vi "CCE RRMA P03 SubVI07.vi"(11 "array":dbl[](array[numeric])) -> (3 "normalizado":dbl[](array[numeric]))   [LabVIEW 2020]
doc: "Ceballos Conde Emanuel Rodríguez Ramírez Miguel Ángel 4MV6 Sistemas de visión artificial 2022/1\neste vi normaliza arreglos como vectores"
panel:
  # "Ceballos Conde Emanuel\nRodríguez Ramírez Miguel Ángel\n4MV6\nSistemas de visión artificial\n2022/1"
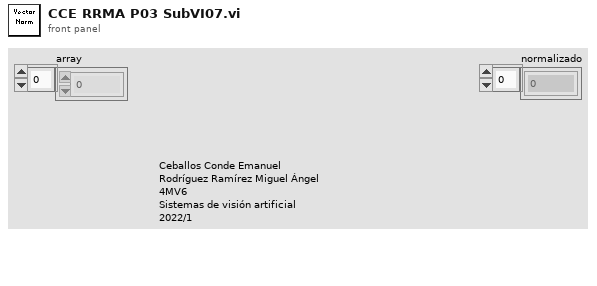
[diagram p1: front panel]
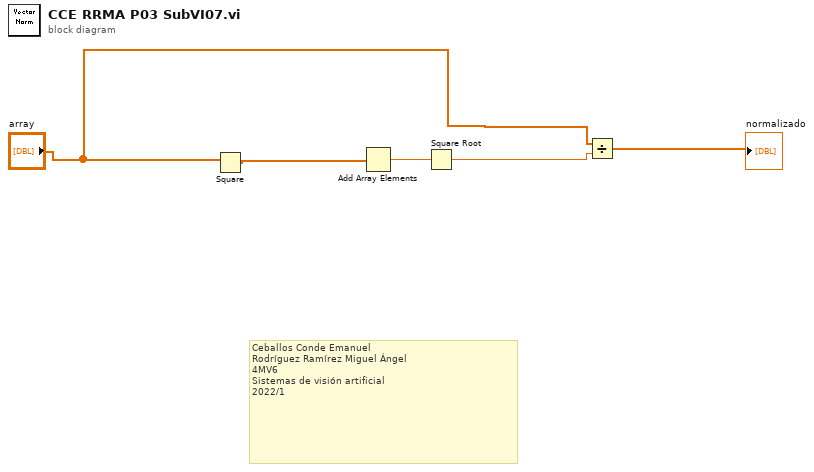
[diagram p0: block diagram]
diagram:
  # "Ceballos Conde Emanuel\nRodríguez Ramírez Miguel Ángel\n4MV6\nSistemas de visión artificial\n2022/1"
  n1 = Square(x="array") -> (x^2=w4:dbl[])
  n2 = Add Array Elements(numeric array=w4) -> (sum=w5:dbl)
  n3 = Square Root(x=w5) -> (sqrt(x)=w2:dbl)
  n4 = Divide(x="array", y=w2) -> (x/y=→"normalizado":dbl[])
